vi "Get RemIO UI Ref.vi"(8 "error in (no error)":errorcluster, 11 "11120 in":refnum<class "11120.lvclass">) -> (0 "error out":errorcluster, 2 "VI Refnum":refnum<vi>, 3 "11120 out":refnum<class "11120.lvclass">)   [LabVIEW 2016, in "Modules.lvlib" / "11120.lvclass"]
uses:
  11120.lvclass
  RemIO Module/RemIO Module.lvclass
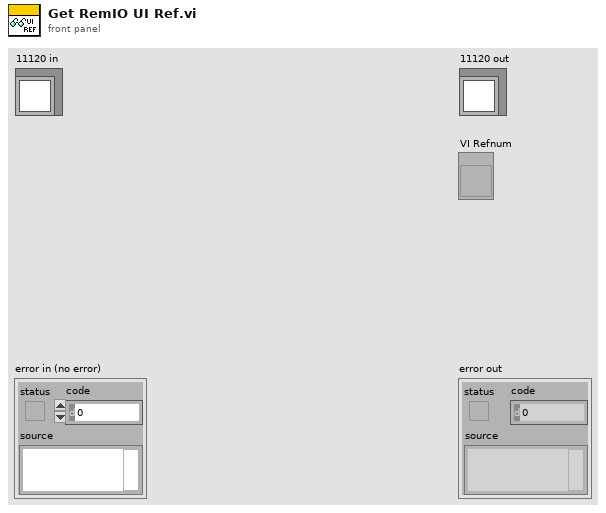
[diagram p1: front panel]
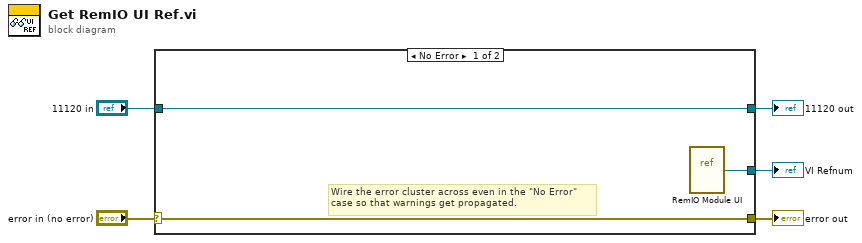
[diagram p0: block diagram]
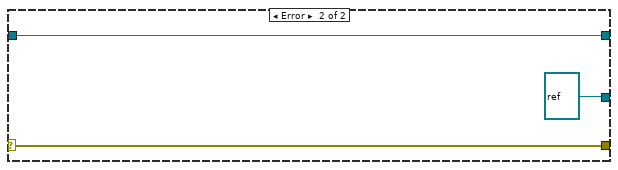
[diagram p2: hidden frame]
diagram:
  n1 = case shown="No Error" "error in (no error)" {
    selector: "error in (no error)" -> [w7 w11]
    tunnel: [w7 w11] -> w3
    tunnel: [w8 w10] -> w1
    tunnel: "11120 in" -> [w8 w10]
    tunnel: [w6 refnum<vi> refnum] -> w5
    frame No Error {
      # "Wire the error cluster across even in the \"No Error\"\ncase so that warnings get propagated."
      n2 = vi-ref "RemIO Module UI.vi"() -> (w6:refnum<vi>)
    }
    frame Error {
    }
  }
  "error out" <- w3
  "11120 out" <- w1
  "VI Refnum" <- w5
